vi "ShotInterception.vi"(5 "Ally?":bool, 7 "BestY":dbl, 8 "error in (no error)":errorcluster, 9 "Game":refnum<class "Game.lvclass">, 10 "Point":dbl[](array[numeric]), 11 "object in":refnum<class "Utilities.lvclass">) -> (0 "error out":errorcluster, 2 "Evaluation":dbl, 3 "object out":refnum<class "Utilities.lvclass">)   [LabVIEW 2023, in "Utilities.lvclass"]
uses:
  Utilities.lvclass
  Game_class/Game.lvclass
  Game_class/Game.lvclass/Game.ctl
  Team_class/Team.lvclass/Team.ctl
  Referee_class/Referee.lvclass/Referee.ctl
  Field_class/Field.lvclass/Field.ctl
  Robot_class/Robot.lvclass/Robot.ctl
  Object_class/Object.lvclass/Object.ctl
  <vilib>/Analysis/coordinate.llb/2D Cartesian Coordinate Shift (Scalar).vi
  <vilib>/Analysis/coordinate.llb/2D Cartesian Coordinate Rotation (Scalar).vi
  Robot_class/Read id.vi
  Object_class/Read position(x,y).vi
  Game_class/Read DefensiveTeam.vi
  Game_class/Read Referee.vi
  Game_class/Read EnemyRef.vi
  Game_class/Read Utilities.lvclass.vi
  Game_class/Read FieldRef.vi
  Game_class/Read NewParameters.vi
  Field_class/Read enemyGoalPosition.vi
  Field_class/Read ourGoalPosition.vi
  Team_class/Read RobotRef.vi
  Referee_class/Read our_goalie_id.vi
  Referee_class/Read enemy_goalie_id.vi
  Enemy_class/Enemy.lvclass
  C:/Users/ebert/Desktop/roboime/SSL_AI/Team_class/Team.lvclass
  Ally_class/Ally.lvclass
  Robot_class/Robot.lvclass
  C:/Users/ebert/Desktop/roboime/SSL_AI/Object_class/Object.lvclass
  Referee_class/Referee.lvclass
  Field_class/Field.lvclass
  <vilib>/Analysis/NI_AALPro.lvlib
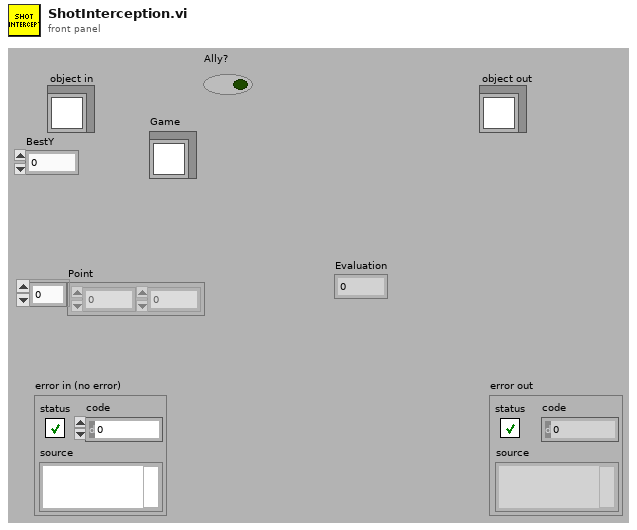
[diagram p1: front panel]
types:
  T1 = typedef "NewParameters.ctl" = cluster{"PenaltyDistance":dbl, "DistanceAttackerToBackBall":dbl, "Division":enum16{"Div B", "Div A"}, "DistanceToAvoidyEnemyRobot":dbl, "BallPlacementDistance":dbl, "DisatanceBehindBallToStealBall":dbl, "MaxDistanceToPositionKickoff":dbl, "BlockEnemyTarget":bool, "MaxStopVAng":dbl, "DistanceMarkerToEnemy":dbl, "IgnoreDribblerContact":bool, "DistanceToBeginEnemyPosession":dbl, "GoToBallWhenEnemyNotMoving":bool, "EnemyDistanceToReduceVelocity":dbl, "TurnOnEnemyDistanceToReduceVelocity":bool, "EnemyDistanceToShootOutBall":dbl, "DefenseKickBall":bool, "MoreKickToGoal? (0-0.3)":dbl, "ChipKickInEnemyField":bool, "ShootOutRobotId":dbl, "FieldLenghtDenominatorInShootOut":dbl, "AdjustPositionInBallPlacement":bool, "PowerGodPass":dbl, "VelocityAbortEnemyPos":dbl, "MaxDistToBeginPass":dbl, "MinDistToBeginPass":dbl, "VelocityInDirects":dbl, "BadDribblerIDs":i32[], "NewKickToDistanceAroundBall":dbl, "PowerAvoidColisionMarker":dbl, "DistanceToAvoidColisionMarker":dbl, "AvoidBallKick":dbl, "DistanceTryKick":dbl, "SuicideKickDIstance":dbl, "AdjustFirstKickDistance":dbl, "AvoidAimLessKick":dbl, "DistanceToAvoidyEnemyShootRobot ":dbl, "NumberOfMarkers":dbl, "PotField":bool, "PIDLateral":bool, "MinDistanceFirstKickX":dbl, "MinDistanceFirstKickY":dbl, "FractionOfDistToTouchGround\nAfterChipKick":dbl, "FractionOfKickxWhen\nComposedWithKickz":dbl, "Style":T2, "MoveInTurnState":bool, "DistFromEnemyToConsider\nMoveInTurnState":dbl, "CascadePID":bool, "TurnAroundParameters":cluster{"Radius":dbl, "Multiplier":dbl, "ChordAngle":dbl}, "SafeDriveVel":dbl, "DistanceToGoToBackBall":dbl, "minDistanceToNotFinish\nEnemyPossession":dbl, "OneTouchShot":cluster{"angleFactor":dbl, "maxAngle":dbl, "Attack":bool, "Defense":bool}, "OpenAngleToGoal":cluster{"minAngle":dbl, "maxAngle":dbl, "minEvaluation":dbl}, "ShotInterception":cluster{"shotSpeed":dbl, "minEnemySpeed":dbl, "maxEnemySpeed":dbl, "minEvaluation":dbl}, "AllyTeamArray":T3[], "maxDefendersNumber":i32, "Zone":cluster{"GuardPositionArray":dbl[][], "ZoneMidField":dbl[], "CenterForwardWidth":dbl}, "MinEvaluationToShoot":dbl, "PassInterception":cluster{"maxPassSpeed":dbl, "minPassSpeed":dbl, "minEnemySpeed":dbl, "chipPassDistance":dbl, "chipPassEvaluation":dbl, "minEvaluation":dbl, "maxEnemySpeed":dbl}, "PassDistance":cluster{"maxDistance":dbl, "minDistance":dbl}, "receiverSpeed":dbl, "maxBallSpeed":dbl, "slackTime":dbl, "Turning radius":dbl, "Turning v_ang":dbl, "AlignError":cluster{"Distance":dbl, "Orientation":dbl, "V_norm(m/s)":dbl, "V_ang (rad/s)":dbl}, "RobotRadius":dbl, "KickerDistance":dbl, "keeper angle  to cover goalpost":dbl}
  T2 = typedef "Style.ctl" = enum16{"Insanity", "Offensive", "Defensive"}
  T3 = typedef "AllyTeam.ctl" = enum16{"Keeper", "Defender", "Attacker"}
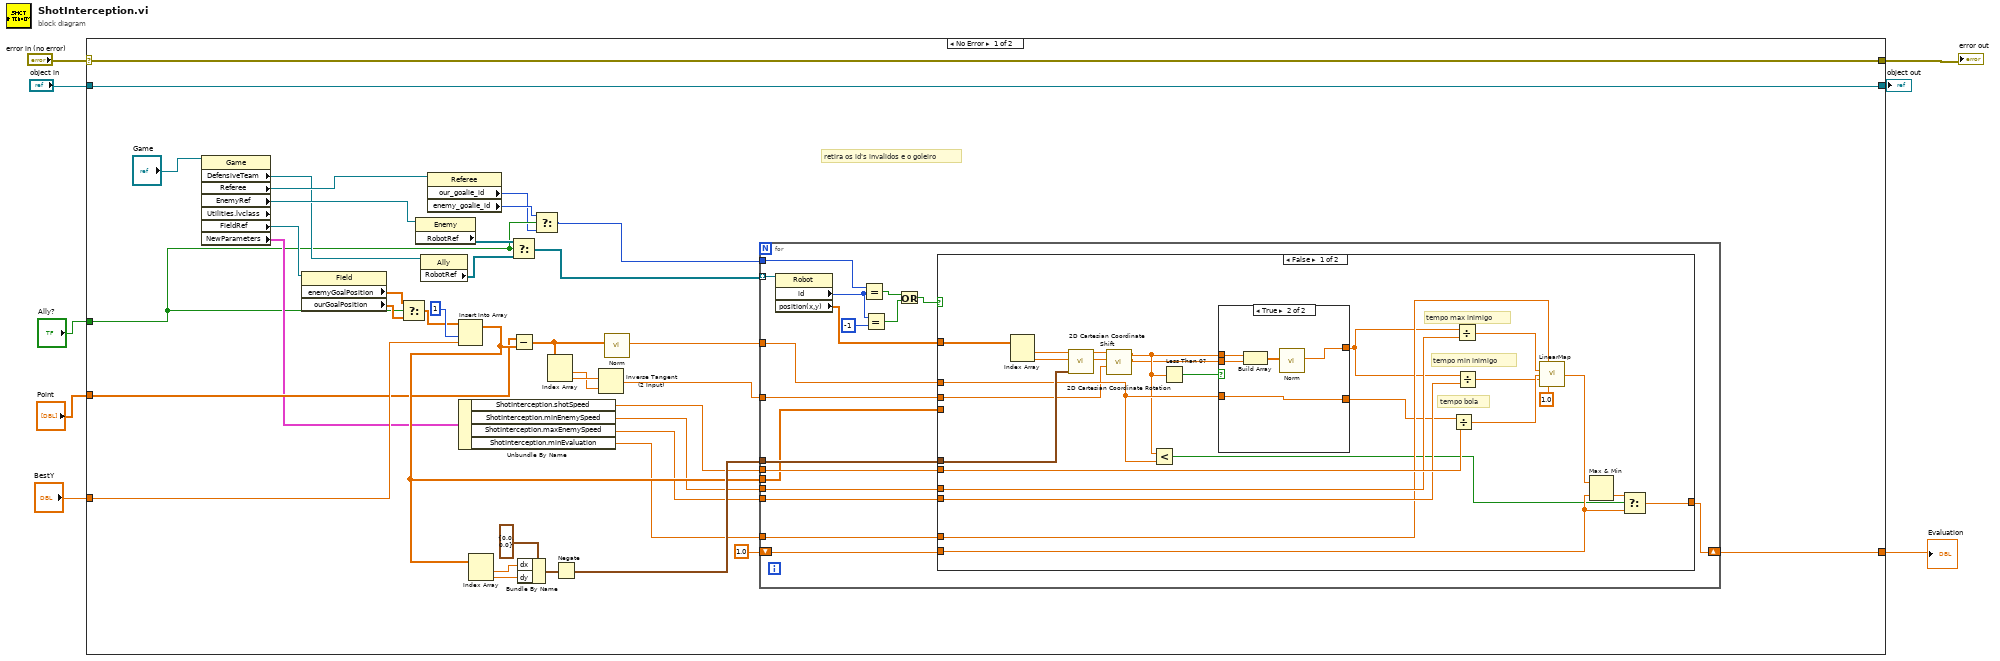
[diagram p0: block diagram]
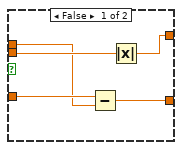
[diagram p2: hidden frame]
diagram:
  n1 = case shown="No Error" "error in (no error)" {
    selector: "error in (no error)" -> [w46 w103]
    tunnel: [w46 w103] -> w7
    tunnel: [w45 w102] -> w5
    tunnel: "object in" -> [w45 w102]
    tunnel: "BestY" -> [w20 _]
    tunnel: "Point" -> [w19 _]
    tunnel: "Ally?" -> [w12 _]
    tunnel: [w18 _] -> w1
    frame No Error {
      # "retira os id's invalidos e o goleiro"
      n2 = property class="Game" props=["DefensiveTeam", "Referee", "EnemyRef", "Utilities.lvclass", "FieldRef", "NewParameters"](reference="Game") -> ("DefensiveTeam"=w14:refnum<class "Ally.lvclass">, "Referee"=w42:refnum<class "Referee.lvclass">, "EnemyRef"=w43:refnum<class "Enemy.lvclass">, "FieldRef"=w30:refnum<class "Field.lvclass">, "NewParameters"=w17:T1)  [unwired: 1 in, 3 out]
      n3 = property class="Field"(reference=w30) -> ("enemyGoalPosition"=w26:dbl[], "ourGoalPosition"=w25:dbl[])  [unwired: 1 in, 2 out]
      n4 = Select(t=w26, s=w12, f=w25) -> (s? t:f=w27:dbl[])
      n5 = property class="Enemy"(reference=w43) -> ("RobotRef"=w15:refnum<class "Robot.lvclass">[])  [unwired: 1 in, 2 out]
      n6 = property class="Ally"(reference=w14) -> ("RobotRef"=w13:refnum<class "Robot.lvclass">[])  [unwired: 1 in, 2 out]
      n7 = property class="Referee"(reference=w42) -> ("our_goalie_id"=w10:i32, "enemy_goalie_id"=w11:i32)  [unwired: 1 in, 2 out]
      n8 = Insert Into Array(array=w27, index=1, new element=w20) -> (w28:dbl[])
      n9 = Unbundle By Name(w17) -> ("ShotInterception.shotSpeed"=w24:dbl, "ShotInterception.minEnemySpeed"=w23:dbl, "ShotInterception.maxEnemySpeed"=w22:dbl, "ShotInterception.minEvaluation"=w21:dbl)
      n10 = Index Array(array=w28) -> (element #1=w37:dbl, element #2=w36:dbl)  [unwired: 2 in]
      n11 = Select(t=w15, s=w12, f=w13) -> (s? t:f=w16:refnum<class "Robot.lvclass">[])
      n12 = Subtract(x=w19, y=w28) -> (x-y=w35:dbl[])
      n13 = Bundle By Name(cluster=cluster{"dx":dbl, "dy":dbl} {"dx"=0.0, "dy"=0.0} ("shift"), "dx"=w37, "dy"=w36) -> (w32:cluster{"dx":dbl, "dy":dbl})
      n14 = Select(t=w11, s=w12, f=w10) -> (s? t:f=w9:i32)
      n15 = Index Array(array=w35) -> (element #1=w40:dbl, element #2=w41:dbl)  [unwired: 2 in]
      n16 = Negate(x=w32) -> (-x=w31:cluster{"dx":dbl, "dy":dbl})
      n17 = Inverse Tangent (2 Input)(1:w40, 2:w41) -> (0:w39:dbl)
      n18 = call "Norm.vi"("2D vector"=w35) -> ("Modulo"=w34:dbl)  [unwired: 8 in, 2 out]
      n19 = for {
        tunnel: w16 -> [w64] mode=indexing
        tunnel: w9 -> [w50]
        tunnel: w39 -> [w63]
        tunnel: w31 -> [w61]
        tunnel: w34 -> [w60]
        tunnel: w24 -> [w59]
        shift-right: [w57] -> w18
        shift-left: 1.0 ("Numeric") -> [w58]
        tunnel: w28 -> [w56]
        tunnel: w23 -> [w55]
        tunnel: w22 -> [w54]
        tunnel: w21 -> [w53]
        n20 = property class="Robot"(reference=w64) -> ("id"=w51:i32, "position(x,y)"=w62:dbl[])  [unwired: 1 in, 2 out]
        n21 = Equal?(x=w50, y=w51) -> (x = y?=w49:bool)
        n22 = Equal?(x=w51, y=-1 ("x")) -> (x = y?=w48:bool)
        n23 = Or(x=w49, y=w48) -> (x .or. y?=w47:bool)
        n24 = case shown="False" w47 {
          tunnel: w63 -> [w82 _]
          tunnel: w62 -> [w88 _]
          tunnel: w61 -> [w90 _]
          tunnel: w60 -> [w86 _]
          tunnel: w59 -> [w87 _]
          tunnel: w58 -> [w83 w101]
          tunnel: [w89 w101] -> w57
          tunnel: w56 -> [_ _]
          tunnel: w55 -> [w85 _]
          tunnel: w54 -> [w84 _]
          tunnel: w53 -> [w81 _]
          frame False {
            # "tempo bola"
            # "tempo min inimigo"
            # "tempo max inimigo"
            n25 = Index Array(array=w88) -> (element #1=w70:dbl, element #2=w69:dbl)  [unwired: 2 in]
            n26 = call-poly <vilib>:"2D Cartesian Coordinate Shift.vi"("shift"=w90, "y"=w69, "x"=w70) -> ("y out"=w67:dbl, "x out"=w68:dbl)  [unwired: 6 in, 1 out]
            n27 = call-poly <vilib>:"2D Cartesian Coordinate Rotation.vi"("theta"=w82, "y"=w67, "x"=w68) -> ("y out"=w65:dbl, "x out"=w66:dbl)  [unwired: 6 in, 1 out]
            n28 = Less?(x=w66, y=w86) -> (x < y?=w79:bool)
            n29 = Less Than 0?(x=w66) -> (x < 0?=w80:bool)
            n30 = case shown="True" w80 {
              tunnel: w66 -> [w91 w98]
              tunnel: w65 -> [w94 w96]
              tunnel: [w93 w100] -> w76
              tunnel: w86 -> [w92 w99]
              tunnel: [w95 w99] -> w75
              frame False {
                n31 = Subtract(x=w92, y=w91) -> (x-y=w95:dbl)
                n32 = Absolute Value(x=w94) -> (abs(x)=w93:dbl)
              }
              frame True {
                n33 = Build Array(w98, w96) -> (w97:dbl[])
                n34 = call "Norm.vi"("2D vector"=w97) -> ("Modulo"=w100:dbl)  [unwired: 8 in, 2 out]
              }
            }
            n35 = Divide(x=w75, y=w87) -> (x/y=w78:dbl)
            n36 = Divide(x=w76, y=w85) -> (x/y=w74:dbl)
            n37 = Divide(x=w76, y=w84) -> (x/y=w73:dbl)
            n38 = call "LinearMap.vi"("MaxY"=w81, "MaxX"=w74, "X"=w78, "MinX"=w73, "MinY"=1.0) -> ("Y"=w72:dbl)  [unwired: 8 in, 2 out]
            n39 = Max & Min(x=w72, y=w83) -> (min(x,y)=w71:dbl)  [unwired: 1 out]
            n40 = Select(t=w71, s=w79, f=w83) -> (s? t:f=w89:dbl)
          }
          frame True {
          }
        }
      }
    }
    frame Error {
    }
  }
  "error out" <- w7
  "object out" <- w5
  "Evaluation" <- w1
